vi "Extend_pulse.vi"(10 "reset":bool, 11 "limit":u16) -> (3 "pulse":bool)   [LabVIEW 2017]
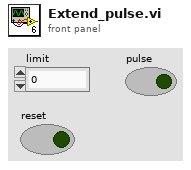
[diagram p1: front panel]
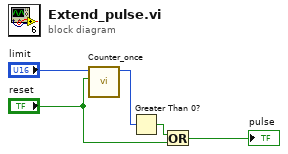
[diagram p0: block diagram]
diagram:
  n1 = call "Counter_once.vi"("reset"="reset", "limit"="limit") -> ("count"=w2:u16)  [unwired: 9 in]
  n2 = Greater Than 0?(x=w2) -> (x > 0?=w3:bool)
  n3 = Or(x=w3, y="reset") -> (x .or. y?=→"pulse":bool)
